vi "MENU6.vi"   [LabVIEW 2012, in "Lazyboots Menu Tool Launch.lvlib"]
uses:
  _Library/Lazyboots Menu Tool Launch.lvlib
  <vilib>/Utility/config.llb/NI_LVConfig.lvlib
  <vilib>/Utility/config.llb/Read Key (String).vi
panel:
  # "Launching..."
types:
  T1 = enum32{"Invalid", "Standard", "Closed", "Hidden", "Minimized", "Maximized"}
  T2 = typedef "NI_LVConfig.lvlib/Config Data RefNum.ctl" = refnum<k1>
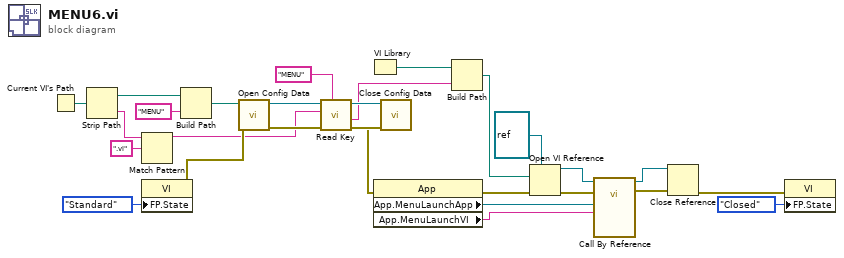
[diagram p0: block diagram]
diagram:
  n1 = Current VI's Path() -> (path=w17:path)
  n2 = Strip Path(path=w17) -> (stripped path=w16:path, name=w6:string)
  n3 = Match Pattern(string=w6, regular expression=".vi") -> (before substring=w5:string)  [unwired: 4 out]
  n4 = property class="VI"("FP.State"=T1."Standard" ("Front Panel Window:State")) -> (error out=w8:errorcluster)  [unwired: 2 in, 1 out]
  n5 = Build Path(base path=w16, name or relative path="MENU") -> (appended path=w14:path)
  n6 = call <vilib>:"Open Config Data.vi"("error in (no error)"=w8, "configuration file path"=w14) -> ("error out"=w12:errorcluster, "refnum"=w13:T2)  [unwired: 7 in, 1 out]
  n7 = call-poly <vilib>:"Read Key.vi"("section"="MENU", "error in (no error)"=w12, "key"=w5, "refnum"=w13) -> ("error out"=w9:errorcluster, "value"=w2:string, "refnum out"=w10:T2)  [unwired: 2 in, 3 out]
  n8 = VI Library() -> (path=w1:path)
  n9 = call <vilib>:"Close Config Data.vi"("error in (no error)"=w9, "refnum"=w10) -> ("error out"=w7:errorcluster)  [unwired: 1 in, 8 out]
  n10 = property class="App"(error in=w7) -> (error out=w24:errorcluster, "App.MenuLaunchApp"=w22:refnum<vi>, "App.MenuLaunchVI"=w21:string)  [unwired: 1 in, 1 out]
  n11 = Build Path(base path=w1, name or relative path=w2) -> (appended path=w3:path)
  n12 = Open VI Reference(type specifier VI Refnum (for type only)=refnum<vi> refnum, vi path=w3, error in (no error)=w24) -> (vi reference=w26:refnum<vi>, error out=w23:errorcluster)  [unwired: 3 out]
  n13 = call-by-ref "?"(reference=w26, error in=w23, "VI Path"=w21, "Application Reference"=w22) -> (reference out=w20:refnum<vi>, error out=w19:errorcluster)  [unwired: 9 in, 1 out]
  n14 = Close Reference(reference=w20, error in (no error)=w19) -> (error out=w18:errorcluster)
  n15 = property class="VI"(error in=w18, "FP.State"=T1."Closed" ("Front Panel Window:State")) -> ()  [unwired: 1 in, 2 out]
